vi "Untitled 1.vi"() -> ()   [LabVIEW 2014]
uses:
  <vilib>/Instr/_visa.llb/VISA Configure Serial Port (Instr).vi
panel:
  in  "Array":i32[](array[numeric])
  in  "VISA resource name":refnum<visa-resource-name>
  in  "stop":bool
  out "read buffer":string
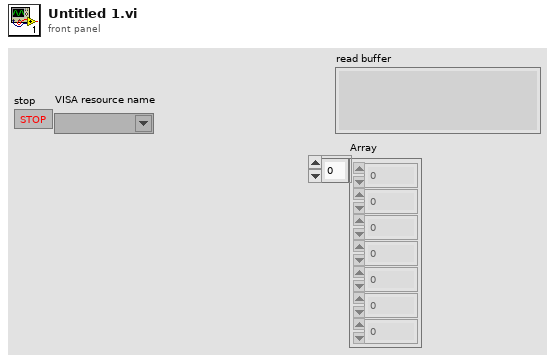
[diagram p1: front panel]
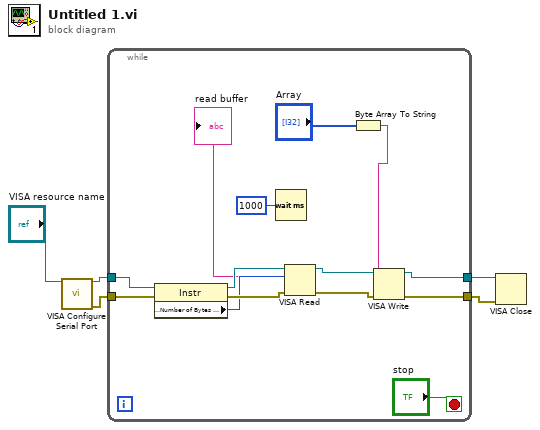
[diagram p0: block diagram]
diagram:
  n1 = call-poly "VISA Configure Serial Port"("VISA resource name"="VISA resource name") -> ("VISA resource name out"=w5:refnum<visa-resource-name>, "error out"=w2:errorcluster)  [unwired: 13 in]
  n2 = while {
    tunnel: w2 -> [w12]
    tunnel: [w15] -> w3
    tunnel: w5 -> [w19]
    tunnel: [w16] -> w4
    stop <- "stop" stop-if-true
    n3 = property class="Instr"(reference=w19, error in=w12) -> (reference out=w18:refnum<visa-resource-name>, error out=w13:errorcluster, "Serial Settings:Number of Bytes at Serial Port"=w11:u32)
    n4 = Wait (ms)(milliseconds to wait=u32 1000) -> ()  [unwired: 1 out]
    n5 = VISA Read(VISA resource name=w18, byte count=w11, error in (no error)=w13) -> (VISA resource name out=w17:refnum<visa-resource-name>, read buffer=→"read buffer":string, error out=w14:errorcluster)  [unwired: 1 out]
    n6 = Byte Array To String(unsigned byte array="Array") -> (string=w8:string)
    n7 = VISA Write(VISA resource name=w17, write buffer=w8, error in (no error)=w14) -> (VISA resource name out=w16:refnum<visa-resource-name>, error out=w15:errorcluster)  [unwired: 1 out]
  }
  n8 = VISA Close(VISA resource name=w4, error in (no error)=w3) -> ()  [unwired: 1 out]
